vi "Split 16xI16 to 8xI16.vi"(0 "data in":i16[](array[numeric])=[0, 0, 0, 0, 0, 0, 0, 0, 0, 0, 0, 0, 0, 0, 0, 0], 2 "reset":bool, 5 "input valid":bool, 12 "ready for output (T)":bool=TRUE) -> (4 "data out":i16[](array[numeric]), 6 "output valid":bool, 14 "ready for input":bool)   [LabVIEW 2018, in "Streaming FPGA.lvlib"]
doc: "Splits an array of 16 I16 elements to multiple arrays of 8 I16 elements. One data input generates two data outputs."
uses:
  Streaming FPGA.lvlib
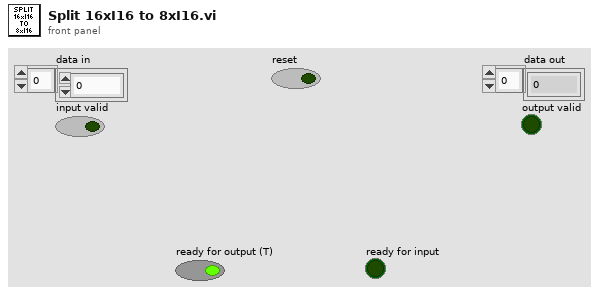
[diagram p1: front panel]
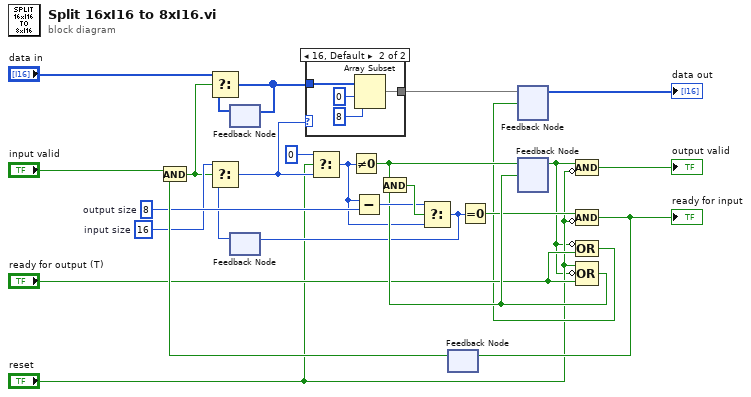
[diagram p0: block diagram]
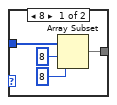
[diagram p2: hidden frame]
diagram:
  w22 = u16 8  # output size
  w10 = u16 16  # input size
  n1 = feedback #1() -> (w13:i16[])  [unwired: 1 in]
  n2 = feedback #2() -> (w20:u16)  [unwired: 1 in]
  n3 = feedback #3() -> (w26:bool)  [unwired: 1 in]
  n4 = And(x="input valid", y=w26) -> (x .and. y?=w8:bool)
  n5 = Select(t="data in", s=w8, f=w13) -> (s? t:f=w12:i16[])
  n6 = Select(t=w10, s=w8, f=w20) -> (s? t:f=w16:u16)
  n7 = feedback-in #1(w12) -> ()
  n8 = case shown="16, Default" w16 {
    tunnel: w12 -> [w30 w34]
    tunnel: [w27 w31] -> w25
    frame 8 {
      n9 = Array Subset(array=w30, index=8, length=8) -> (w27:i16[])
    }
    frame 16, Default {
      n10 = Array Subset(array=w34, index=0, length=8) -> (w31:i16[])
    }
  }
  n11 = Select(t=u16 0, s="reset", f=w16) -> (s? t:f=w14:u16)
  n12 = Not Equal To 0?(x=w14) -> (x != 0?=w24:bool)
  n13 = Subtract(x=w14, y=w22) -> (x-y=w21:u16)
  n14 = feedback #4() -> (→"data out":i16[])  [unwired: 1 in]
  n15 = feedback #5() -> (w1:bool)  [unwired: 1 in]
  n16 = Compound Arithmetic op=AND(w1, invert "reset") -> (→"output valid":bool)
  n17 = Compound Arithmetic op=OR(invert w1, "ready for output (T)") -> (w3:bool)
  n18 = feedback-in #4(w25, w3) -> ()
  n19 = Compound Arithmetic op=OR("reset", invert w1, "ready for output (T)") -> (w19:bool)
  n20 = And(x=w24, y=w19) -> (x .and. y?=w23:bool)
  n21 = Select(t=w21, s=w23, f=w14) -> (s? t:f=w18:u16)
  n22 = feedback-in #2(w18) -> ()
  n23 = Equal To 0?(x=w18) -> (x = 0?=w17:bool)
  n24 = feedback-in #5(w24, w19) -> ()
  n25 = Compound Arithmetic op=AND(w17, invert "reset") -> (w6:bool)
  "ready for input" <- w6
  n26 = feedback-in #3(w6) -> ()
